vi "Get Red.vi"(8 "error in (no error)":errorcluster, 11 "Color in":refnum<class "Color.lvclass">) -> (0 "error out":errorcluster, 2 "Red":u8, 3 "Color out":refnum<class "Color.lvclass">)   [LabVIEW 2020, in "RPI.SenseHat.Display.lvlib" / "Color.lvclass"]
doc: "Returns the red component."
uses:
  Color.lvclass
  Color.lvclass/Color.ctl
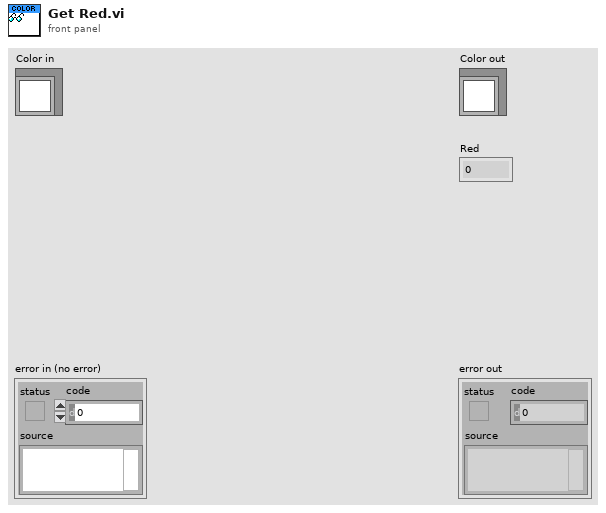
[diagram p1: front panel]
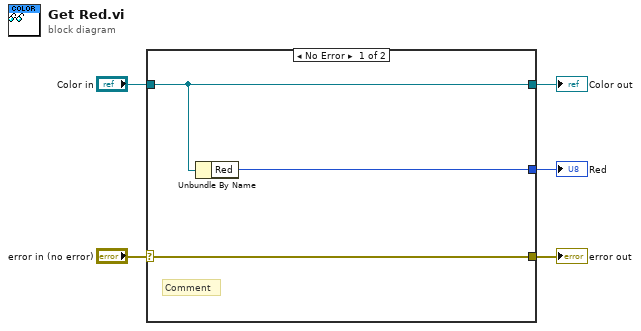
[diagram p0: block diagram]
diagram:
  n1 = case shown="No Error" "error in (no error)" {
    selector: "error in (no error)" -> [w8 w9]
    tunnel: [w8 w9] -> w4
    tunnel: [w7 w10] -> w2
    tunnel: "Color in" -> [w7 w10]
    tunnel: [w6 _] -> w1
    frame No Error {
      # "Comment"
      n2 = Unbundle By Name(w7) -> ("Red"=w6:u8)
    }
    frame Error {
    }
  }
  "error out" <- w4
  "Color out" <- w2
  "Red" <- w1
